vi "Mark as Set.vi"(10 "Field name":string, 11 "Object Type in":refnum<class "Object Type Base.lvclass">) -> (3 "Object Type out":refnum<class "Object Type Base.lvclass">)   [LabVIEW 2019, in "Electronic Datasheet.lvlib" / "Object Type Base.lvclass"]
uses:
  Object Type Base.lvclass
  Object Type Base.lvclass/Object Type Base.ctl
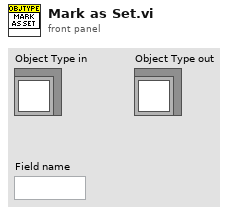
[diagram p1: front panel]
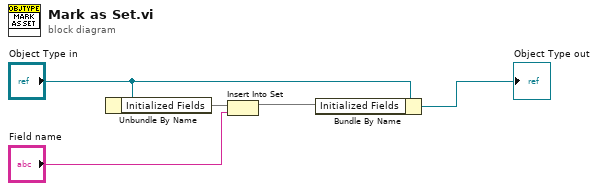
[diagram p0: block diagram]
diagram:
  n1 = Unbundle By Name("Object Type in") -> ("Initialized Fields"=w5:set{string})
  n2 = Insert Into Set(10:"Field name", 11:w5) -> (3:w1:set{string})  [unwired: 1 out]
  n3 = Bundle By Name(cluster="Object Type in", "Initialized Fields"=w1) -> (→"Object Type out":refnum<class "Object Type Base.lvclass">)
